vi "test_merge.vi"(1 "Control":T1, 2 "Status":T2) -> (0 "Cluster":T3)   [LabVIEW 2019]
uses:
  test_cluster.ctl
  Control.ctl
  Staus.ctl
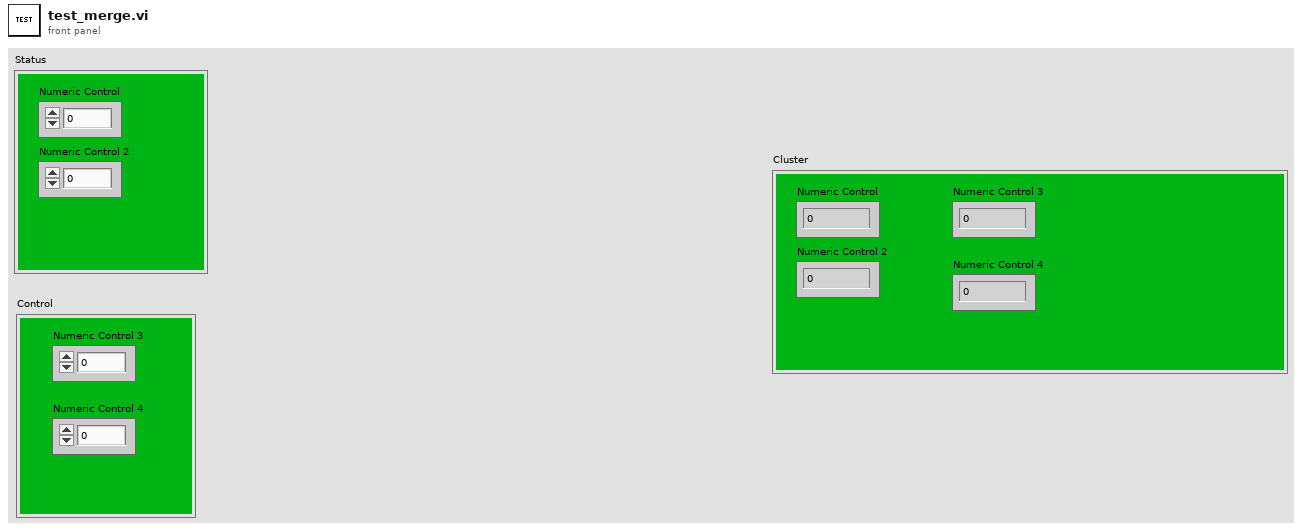
[diagram p1: front panel]
types:
  T1 = typedef "Staus.ctl" = cluster{"Numeric Control 3":dbl, "Numeric Control 4":dbl}
  T2 = typedef "Control.ctl" = cluster{"Numeric Control":dbl, "Numeric Control 2":dbl}
  T3 = typedef "test_cluster.ctl" = cluster{"Numeric Control":dbl, "Numeric Control 2":dbl, "Numeric Control 3":dbl, "Numeric Control 4":dbl}
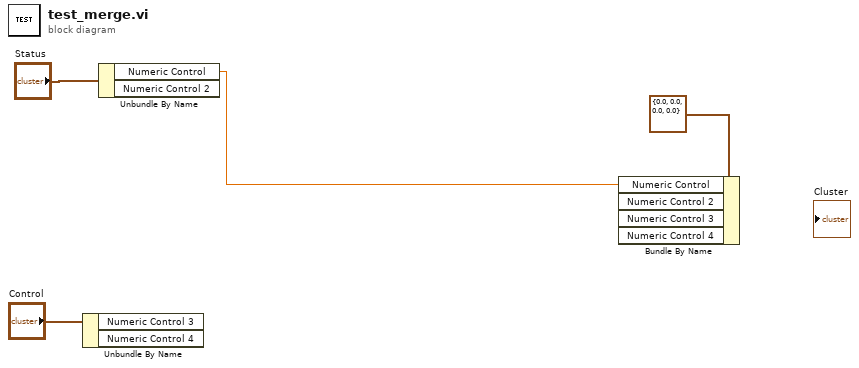
[diagram p0: block diagram]
diagram:
  n1 = Unbundle By Name("Control") -> ()  [unwired: 2 out]
  n2 = Unbundle By Name("Status") -> ("Numeric Control"=w1:dbl)  [unwired: 1 out]
  n3 = Bundle By Name(cluster=T3 {"Numeric Control"=0.0, "Numeric Control 2"=0.0, "Numeric Control 3"=0.0, "Numeric Control 4"=0.0} ("Cluster"), "Numeric Control"=w1) -> ()  [unwired: 3 in, 1 out]
